vi "squiggle_write_all.vi"(6 "Init sequence":u8[](array[numeric]), 8 "Error in":errorcluster, 9 "Pulse count":i16[](array[numeric]), 10 "Send init sequence":bool, 11 "I2C interface":T1) -> (0 "Error out":errorcluster)   [LabVIEW 2013]
uses:
  i2c_interface.ctl
  fpga_reference.ctl
  Common/demux_command.ctl
panel:
  in  "Sequence number":u8
  # "Write an I2C command to all six squiggle motor controllers.  If \"Send init sequence\" is false (default), then write the specified \"Pulse count\" values to each axis.  If \"Send init sequence\" is true, then write the same init sequence to every motor."
  # "Locals:"
  # "This remaps the documented motor numbers\nonto the actual wiring arrangement, constrained\nby the flex layout.   The index is the output\naxis and the element is the input axis."
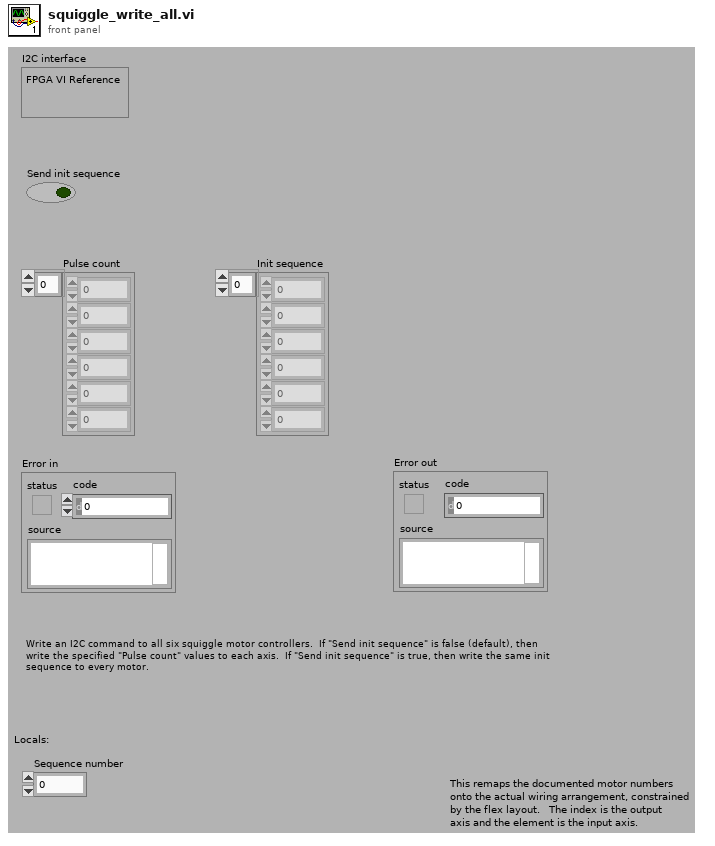
[diagram p1: front panel]
types:
  T1 = typedef "i2c_interface.ctl" = cluster{"FPGA VI Reference":T2}
  T2 = typedef "fpga_reference.ctl" = refnum<k20>
  T3 = typedef "demux_command.ctl" = enum8{"bus_0", "bus_1", "bus_2", "invalid_3", "invalid_4", "drain_fifo", "wait_hard_trigger", "wait_soft_trigger", "trigger_enable"}
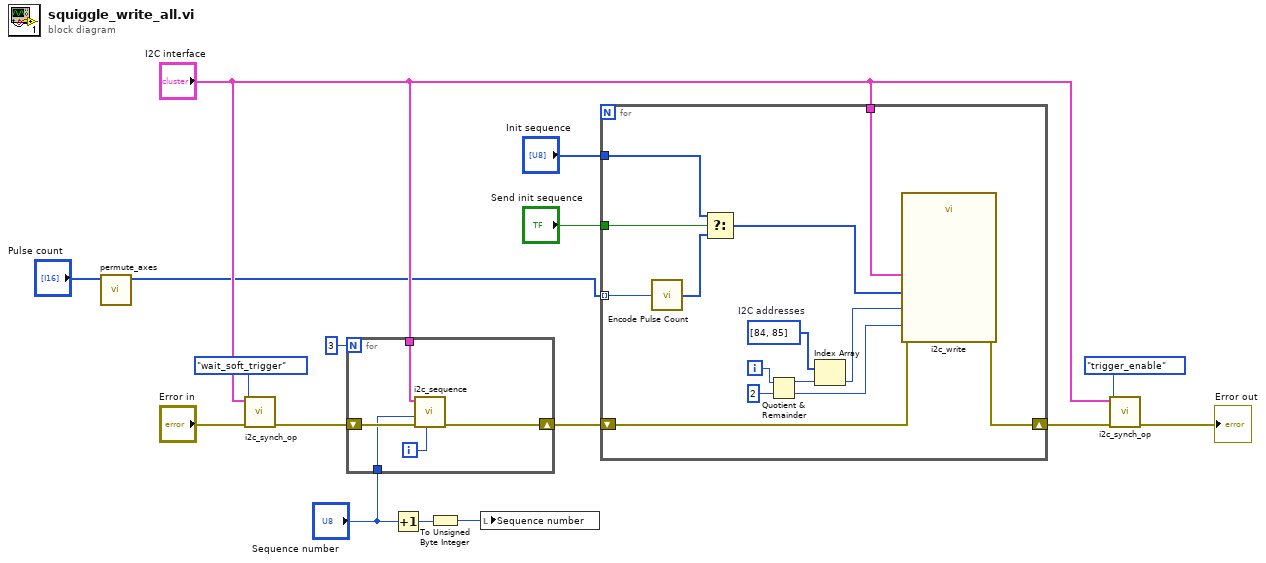
[diagram p0: block diagram]
diagram:
  n1 = call "permute_axes.vi"("Pulse count"="Pulse count") -> ("Result"=w1:i16[])  [unwired: 10 in]
  n2 = call "i2c_synch_op.vi"("error in"="Error in", "Demux command"=demux_command."wait_soft_trigger", "I2C interface"="I2C interface") -> ("error out"=w9:errorcluster)  [unwired: 7 in, 1 out]
  n3 = for {
    N: 3 -> [_]
    shift-right: [w19] -> w6
    shift-left: w9 -> [w21]
    tunnel: "I2C interface" -> [w20]
    tunnel: "Sequence number" -> [w17]
    i -> [w18]
    n4 = call "i2c_sequence.vi"("Bus"=w18, "error in"=w21, "Sequence number"=w17, "I2C interface"=w20) -> ("error out"=w19:errorcluster)  [unwired: 6 in, 1 out]
  }
  n5 = Increment(x="Sequence number") -> (x+1=w5:u8)
  n6 = To Unsigned Byte Integer(number=w5) -> (unsigned 8bit integer=w3:u8)
  n7 = local write "Sequence number"(w3) -> ()
  n8 = for {
    tunnel: "Send init sequence" -> [w33]
    tunnel: w1 -> [w26] mode=indexing
    shift-right: [w34] -> w14
    shift-left: w6 -> [w35]
    tunnel: "Init sequence" -> [w25]
    tunnel: "I2C interface" -> [w24]
    i -> [w30]
    w28 = u8[] [84, 85]  # I2C addresses
    n9 = call "Encode Pulse Count.vi"("Pulse count"=w26) -> ("Array"=w31:u8[])
    n10 = Select(t=w25, s=w33, f=w31) -> (s? t:f=w32:u8[])
    n11 = Quotient & Remainder(x=w30, y=2) -> (x-y*floor(x/y)=w27:i32, floor(x/y)=w23:i32)
    n12 = Index Array(array=w28, index=w27) -> (element=w22:u8)
    n13 = call "i2c_write.vi"("Bus"=w23, "error in"=w35, "Data"=w32, "Address"=w22, "I2C interface"=w24) -> ("error out"=w34:errorcluster)  [unwired: 5 in, 1 out]
  }
  n14 = call "i2c_synch_op.vi"("error in"=w14, "Demux command"=demux_command."trigger_enable", "I2C interface"="I2C interface") -> ("error out"=→"Error out":errorcluster)  [unwired: 7 in, 1 out]
